vi "Log Measurement.vi"(8 "error in (no error)":errorcluster, 10 "Measurement Results":T1, 11 "Json Logger in":refnum<class "Json Logger Client.lvclass">) -> (0 "error out":errorcluster, 3 "Json Logger out":refnum<class "Json Logger Client.lvclass">)   [LabVIEW 2021, in "Json Logger Client.lvclass"]
doc: "The measurement results are formatted as a request body to be passed as a parameter to the Logger service method. This method will be invoked through the created client stub, and the operation will be executed when this VI is called, with a timeout of 300 milliseconds."
uses:
  Json Logger Client.lvclass
  NI-DCPower Measurement/Measurement Results.ctl
  Json Logger Client.lvclass/Json Logger Client.ctl
  stubs/log_measurement_client.lvlib
  NI-DCPower Measurement/NIDCPowerSourceDCVoltage.lvlib
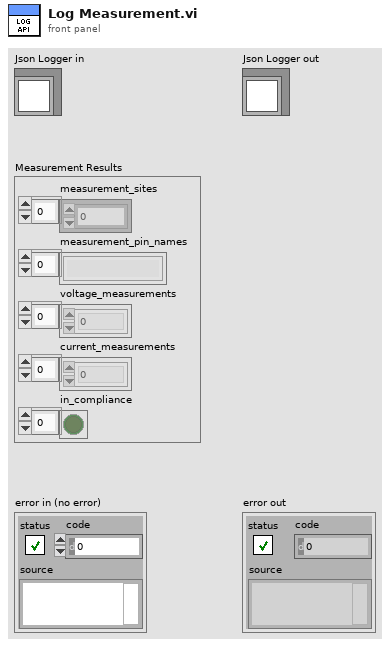
[diagram p1: front panel]
types:
  T1 = typedef "NIDCPowerSourceDCVoltage.lvlib/Measurement Results.ctl" = cluster{"measurement_sites":i32[], "measurement_pin_names":string[], "voltage_measurements":dbl[], "current_measurements":dbl[], "in_compliance":bool[]}
  T2 = typedef "grpc-lvsupport-release.lvlib/grpcId.ctl" = u64
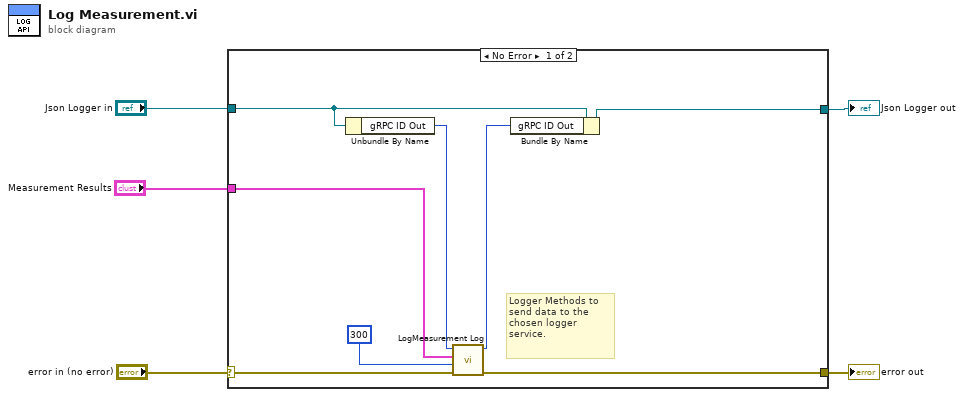
[diagram p0: block diagram]
diagram:
  n1 = case shown="No Error" "error in (no error)" {
    selector: "error in (no error)" -> [w12 w15]
    tunnel: [w13 w15] -> w4
    tunnel: [w9 w14] -> w2
    tunnel: "Json Logger in" -> [w7 w14]
    tunnel: "Measurement Results" -> [w10 _]
    frame No Error {
      # "Logger Methods to send data to the chosen logger service."
      n2 = Unbundle By Name(w7) -> ("gRPC ID Out"=w6:T2)
      n3 = call "LogMeasurement Log.vi"("error in"=w12, "timeout (ms)"=300, "Request Data"=w10, "gRPC ID"=w6) -> ("error out"=w13:errorcluster, "gRPC ID out"=w8:T2)  [unwired: 5 in, 1 out]
      n4 = Bundle By Name(cluster=w7, "gRPC ID Out"=w8) -> (w9:refnum<class "Json Logger Client.lvclass">)
    }
    frame Error {
    }
  }
  "error out" <- w4
  "Json Logger out" <- w2
